vi "MGI Generate Orthonormal Basis.vi"(1 "3 Points":dbl[][](array[numeric]) format="%.2f") -> (0 "3 Basis Vectors":dbl[][](array[numeric]) format="%.2f")   [LabVIEW 2016]
doc: "Generate a set of orthonormal basis vectors from three points given in cartesian coordinates. The basis vectors are found by normalizing:\nw1=p1-p2\nw2=w1 x (p2-p3)\nw3=w1 x w2\n\nAuthored by David A. Moore\nsupport@mooregoodideas.com\nwww.mooregoodideas.com\n\nCopyright (c) 2010, Moore Good Ideas, Inc.\n\nAll rights reserved.\n\nRedistribution and use in source and binary forms, with or without modification, are permitted provided that the following conditions are met:\n\n * Redistributions of source code must retain the above copyright notice, this list of conditions and the following disclaimer.\n * Redistributions in binary form must reproduce the above copyright notice, this list of conditions and the following disclaimer in the documentation and/or other materials provided with the distribution.\n * Neither the name of Moore Good Ideas, Inc. nor the names of its contributors may be used to endorse or promote products derived from this software without specific prior written permission.\n\nTHIS SOFTWARE IS PROVIDED BY THE COPYRIGHT HOLDERS AND CONTRIBUTORS \"AS IS\" AND ANY EXPRESS OR IMPLIED WARRANTIES, INCLUDING, BUT NOT LIMITED TO, THE IMPLIED WARRANTIES OF MERCHANTABILITY AND FITNESS FOR A PARTICULAR PURPOSE ARE DISCLAIMED. IN NO EVENT SHALL THE COPYRIGHT OWNER OR CONTRIBUTORS BE LIABLE FOR ANY DIRECT, INDIRECT, INCIDENTAL, SPECIAL, EXEMPLARY, OR CONSEQUENTIAL DAMAGES (INCLUDING, BUT NOT LIMITED TO, PROCUREMENT OF SUBSTITUTE GOODS OR SERVICES; LOSS OF USE, DATA, OR PROFITS; OR BUSINESS INTERRUPTION) HOWEVER CAUSED AND ON ANY THEORY OF LIABILITY, WHETHER IN CONTRACT, STRICT LIABILITY, OR TORT (INCLUDING NEGLIGENCE OR OTHERWISE) ARISING IN ANY WAY OUT OF THE USE OF THIS SOFTWARE, EVEN IF ADVISED OF THE POSSIBILITY OF SUCH DAMAGE."
uses:
  <vilib>/Analysis/baseanly.llb/Unit Vector (DBL).vi
  <userlib>/_MGI/Matrix & Vector/MGI Cross Product/MGI Cross Product DBL.vi
  <vilib>/Analysis/NI_AALBase.lvlib
panel:
  # "coord1"
  # "coord2"
  # "coord3"
  # "coord1"
  # "coord2"
  # "coord3"
  # "v1"
  # "pt1"
  # "v2"
  # "pt2"
  # "v3"
  # "pt3"
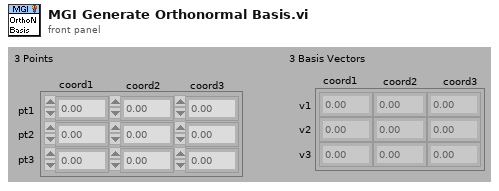
[diagram p1: front panel]
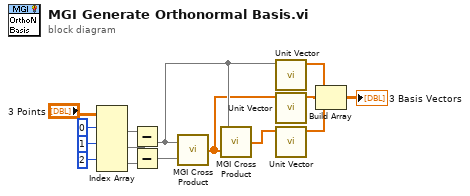
[diagram p0: block diagram]
diagram:
  n1 = Index Array(array="3 Points", index (row) #1=0 ("Index (row)"), index (row) #2=1 ("Index (row)"), index (row) #3=2 ("Index (row)")) -> (element #1=w11:dbl[], element #2=w9:dbl[], element #3=w10:dbl[])  [unwired: 3 in]
  n2 = Subtract(x=w11, y=w9) -> (x-y=w7:dbl[])
  n3 = Subtract(x=w9, y=w10) -> (x-y=w8:dbl[])
  n4 = call-poly <userlib>:"MGI Cross Product.vi"("B[]"=w8, "A[]"=w7) -> ("AxB[]"=w6:dbl[])
  n5 = call-poly <userlib>:"MGI Cross Product.vi"("B[]"=w6, "A[]"=w7) -> ("AxB[]"=w5:dbl[])
  n6 = call-poly <vilib>:"Unit Vector.vi"("Input Vector"=w7) -> ("Unit Vector"=w3:dbl[])  [unwired: 8 in, 2 out]
  n7 = call-poly <vilib>:"Unit Vector.vi"("Input Vector"=w6) -> ("Unit Vector"=w4:dbl[])  [unwired: 8 in, 2 out]
  n8 = call-poly <vilib>:"Unit Vector.vi"("Input Vector"=w5) -> ("Unit Vector"=w2:dbl[])  [unwired: 8 in, 2 out]
  n9 = Build Array(w3, w4, w2) -> (→"3 Basis Vectors":dbl[][])
